vi "Getres_name.vi"(8 "error in (no error)":errorcluster, 11 "OneOfTemplate in":refnum<class "Greeter_res_res_oneof.lvclass">) -> (0 "error out":errorcluster, 2 "Get_Val":string, 3 "OneOfTemplate out":refnum<class "Greeter_res_res_oneof.lvclass">)   [LabVIEW 2019, in "Generated_server.lvlib" / "Greeter_res_res_oneof.lvclass"]
uses:
  Greeter_res_res_oneof.lvclass
  Greeter_res_res_oneof.lvclass/Greeter_res_res_oneof.ctl
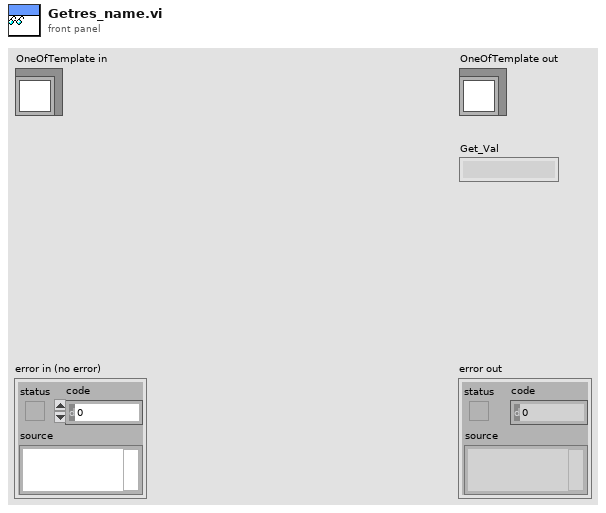
[diagram p1: front panel]
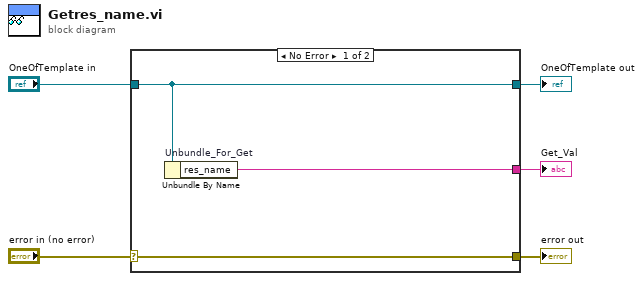
[diagram p0: block diagram]
diagram:
  n1 = case shown="No Error" "error in (no error)" {
    selector: "error in (no error)" -> [w8 w9]
    tunnel: [w8 w9] -> w4
    tunnel: [w7 w10] -> w2
    tunnel: "OneOfTemplate in" -> [w7 w10]
    tunnel: [w6 _] -> w1
    frame No Error {
      n2 = Unbundle By Name "Unbundle_For_Get"(w7) -> ("res_name"=w6:string)
    }
    frame Error {
    }
  }
  "error out" <- w4
  "OneOfTemplate out" <- w2
  "Get_Val" <- w1
